vi "Close Notification.vi"() -> ()   [LabVIEW 2009, in "UI.lvlib"]
uses:
  UI.lvlib
panel:
  in  "Stop":bool
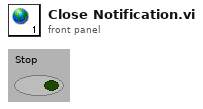
[diagram p1: front panel]
diagram:
